vi "oax_Get Channel Info (DAQmx DSA).vi"(8 "error in (no error)":errorcluster, 9 "Tacho Type":enum16{"Analog Tacho", "Digital Tacho"}(ring), 10 "tachometer channel":tag, 11 "DAQ Config":T4 {"pregain" format="%.2f"; "IEPE" items=["On", "Off", "None"]; "coupling" items=["DC", "AC"]; "engineering units" items=["custom..."=0, "V"=1, "A"=21, "C"=30, "pC"=31, "s"=32, "-"=29, "Pa"=2, "N"=20, "g"=3, "m/s^2"=4, "m/s"=5, "m"=6, "mm/s"=12, "mm"=13, "micron/s"=14, "micron"=15, "in/s^2"=7, "in/s"=8, "in"=9, "mil/s"=10, "mil"=11, "rad/s^2"=16, "rad/s"=17, "rad"=18, "deg/s^2"=26, "deg/s"=27, "deg"=28, "RPM"=22, "cycle/s^2"=23, "Hz"=24, "cycle"=25, "strain"=19]; "sensor sensitivity (mV/EU)" format="%.2f"; "dB reference" format="%.1e"}) -> (0 "error out":errorcluster, 1 "tachometer channel selected":tag, 2 "channel name":string[](array[string]), 3 "channel info":T1[](array[typedef]) {"pregain" format="%.2f"; "weighting filter" items=["Linear", "A-weighting", "B-weighting", "C-weighting", "ITU-R 468-4", "Dolby", "CCITT", "C-message", "Wb", "Wc", "Wd", "We", "Wf", "Wh", "Wj", "Wk", "Wm", "AES17 20 kHz lowpass", "AES17 40 kHz lowpass", "AES17 20 kHz highpass", "AES17 40 kHz highpass"]; "dB reference" format="%^.1e"; "engineering units" items=["custom..."=0, "V"=1, "A"=21, "C"=30, "pC"=31, "s"=32, "-"=29, "Pa"=2, "N"=20, "g"=3, "m/s^2"=4, "m/s"=5, "m"=6, "mm/s"=12, "mm"=13, "micron/s"=14, "micron"=15, "in/s^2"=7, "in/s"=8, "in"=9, "mil/s"=10, "mil"=11, "rad/s^2"=16, "rad/s"=17, "rad"=18, "deg/s^2"=26, "deg/s"=27, "deg"=28, "RPM"=22, "cycle/s^2"=23, "Hz"=24, "cycle"=25, "strain"=19]; "sensor sensitivity" format="%#_5f"}, 4 "tacho channel index":i32, 5 "dul tacho type":enum16{"Analog Tacho", "Digital Tacho"}(ring))   [LabVIEW 2017]
doc: "Configure and organize channel information."
uses:
  <vilib>/addons/Sound and Vibration/Order Analysis/Example Support/sub VIs/OAXML_DSA DAQ Config.ctl
  <vilib>/addons/_NISVFA/_Shared subVIs/Controls/svc_Engineering Units Text Ring.ctl
  <vilib>/addons/_NISVFA/_Shared subVIs/Controls/svc_Channel Info.ctl
  <vilib>/addons/_NISVFA/_Shared subVIs/Controls/svc_Weighting Filter Text Ring.ctl
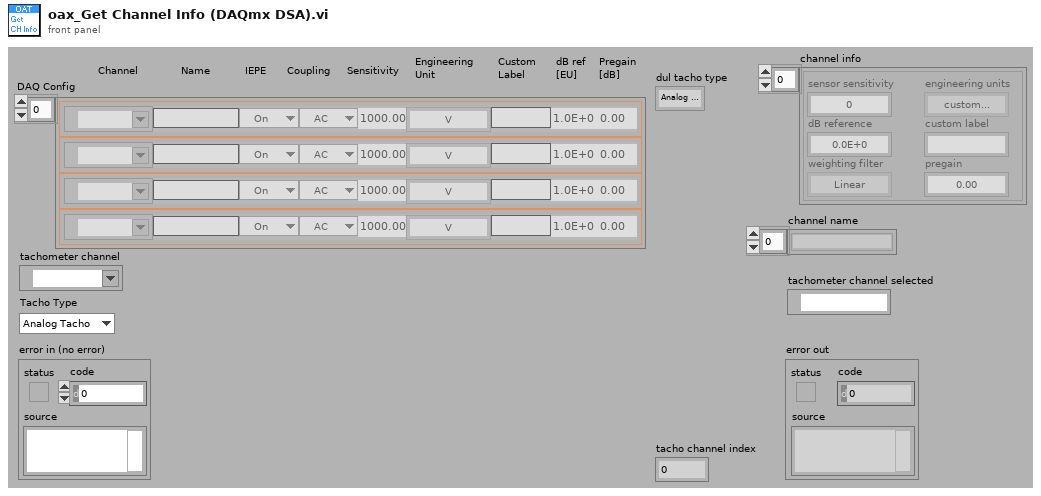
[diagram p1: front panel]
types:
  T1 = typedef "svc_Channel Info.ctl" = cluster{"sensor sensitivity":dbl, "engineering units":T2, "dB reference":dbl, "custom label":string, "weighting filter":T3, "pregain":dbl}
  T2 = typedef "svc_Engineering Units Text Ring.ctl" = u16
  T3 = typedef "svc_Weighting Filter Text Ring.ctl" = u16
  T4 = typedef "OAXML_DSA DAQ Config.ctl" = cluster{"name":string, "channel":tag, "coupling":u16, "dB reference":sgl, "sensor sensitivity (mV/EU)":dbl, "engineering units":T2, "IEPE":u16, "custom label":string, "pregain":sgl}[]
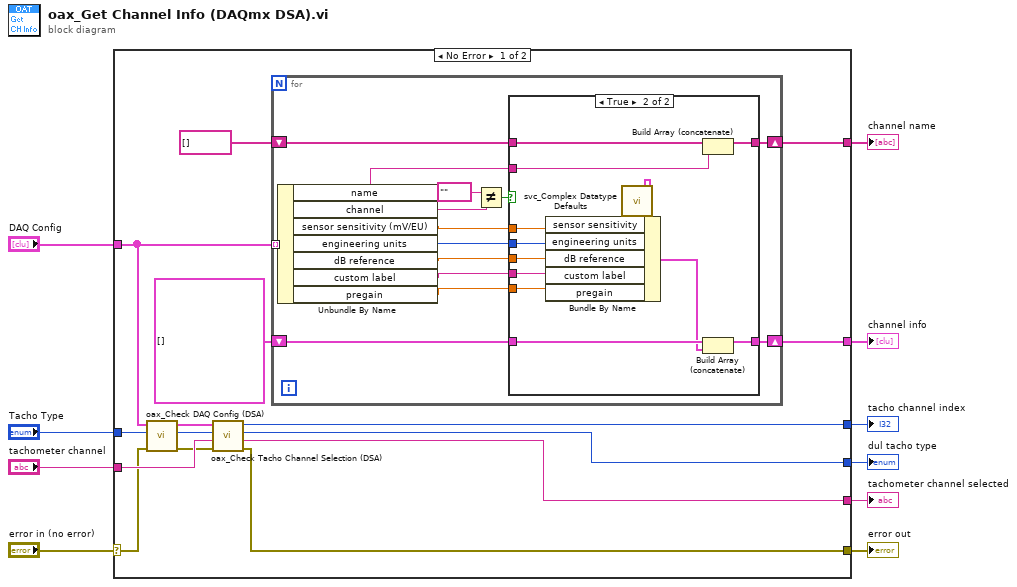
[diagram p0: block diagram]
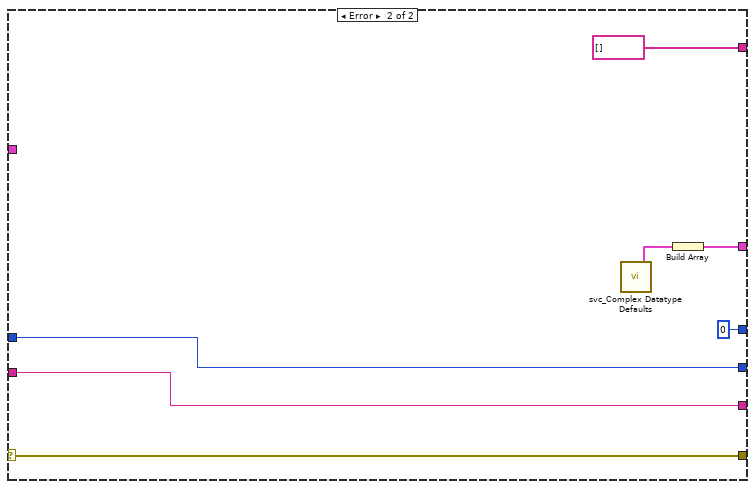
[diagram p3: hidden frame]
diagram:
  n1 = case shown="No Error" "error in (no error)" {
    selector: "error in (no error)" -> [w13 w59]
    tunnel: "DAQ Config" -> [w17 _]
    tunnel: [w24 string[] [] ("channel name")] -> w8
    tunnel: [w23 w54] -> w7
    tunnel: [w21 w59] -> w6
    tunnel: "Tacho Type" -> [w14 w57]
    tunnel: "tachometer channel" -> [w22 w56]
    tunnel: [w20 w56] -> w3
    tunnel: [w19 0 ("tacho channel index")] -> w2
    tunnel: [w18 w57] -> w1
    frame No Error {
      n2 = call <vilib>:"oax_Check DAQ Config (DSA).vi"("error in (no error)"=w13, "Tacho Type"=w14, "DAQ Config"=w17) -> ("error out"=w12:errorcluster, "dup Tacho Type"=w15:enum16{"Analog Tacho", "Digital Tacho"}, "dup DAQ Config"=w16:T4)  [unwired: 6 in]
      n3 = call <vilib>:"oax_Check Tacho Channel Selection (DSA).vi"("error in (no error)"=w12, "tachometer channel"=w22, "tacho type"=w15, "DAQ Config"=w16) -> ("error out"=w21:errorcluster, "tachometer channel selected"=w20:tag, "dul tacho type"=w18:enum16{"Analog Tacho", "Digital Tacho"}, "tacho channel index"=w19:i32)  [unwired: 4 in]
      n4 = for {
        tunnel: w17 -> [w28] mode=indexing
        shift-right: [w31] -> w24
        shift-left: string[] [] ("channel name") -> [w32]
        shift-right: [w29] -> w23
        shift-left: T1[] [] -> [w30]
        n5 = Unbundle By Name(w28) -> ("name"=w33:string, "channel"=w26:tag, "sensor sensitivity (mV/EU)"=w35:dbl, "engineering units"=w39:T2, "dB reference"=w38:sgl, "custom label"=w37:string, "pregain"=w36:sgl)
        n6 = Not Equal?(x=tag "" ("channel"), y=w26) -> (x != y?=w34:bool)
        n7 = case shown="True" w34 {
          tunnel: w35 -> [_ w53]
          tunnel: w39 -> [_ w52]
          tunnel: w38 -> [_ w51]
          tunnel: w37 -> [_ w50]
          tunnel: w36 -> [_ w49]
          tunnel: w33 -> [_ w44]
          tunnel: w32 -> [w40 w45]
          tunnel: [w40 w43] -> w31
          tunnel: w30 -> [w41 w48]
          tunnel: [w41 w46] -> w29
          frame False {
          }
          frame True {
            n8 = call <vilib>:"svc_Complex Datatype Defaults.vi"() -> ("channel info"=w42:T1)  [unwired: 11 in, 8 out]
            n9 = Bundle By Name(cluster=w42, "sensor sensitivity"=w53, "engineering units"=w52, "dB reference"=w51, "custom label"=w50, "pregain"=w49) -> (w47:T1)
            n10 = Build Array (concatenate)(w45, w44) -> (w43:string[])
            n11 = Build Array (concatenate)(w48, w47) -> (w46:T1[])
          }
        }
      }
    }
    frame Error {
      n12 = call <vilib>:"svc_Complex Datatype Defaults.vi"() -> ("channel info"=w55:T1)  [unwired: 11 in, 8 out]
      n13 = Build Array(w55) -> (w54:T1[])
    }
  }
  "channel info" <- w7
  "channel name" <- w8
  "error out" <- w6
  "tachometer channel selected" <- w3
  "tacho channel index" <- w2
  "dul tacho type" <- w1
